vi "Close Tricon.vi"(11 "VISA resource name":refnum<visa-resource-name>="COM3") -> (0 "error out":errorcluster)   [LabVIEW 2018]
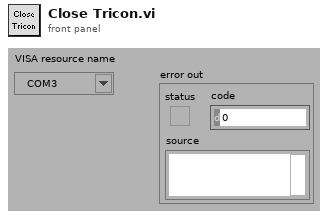
[diagram p1: front panel]
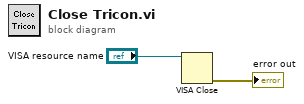
[diagram p0: block diagram]
diagram:
  n1 = VISA Close(VISA resource name="VISA resource name") -> (error out=→"error out":errorcluster)  [unwired: 1 in]
